vi "Serial Send Characters To Arduino.vi"() -> ()   [LabVIEW 2014]
uses:
  <vilib>/Instr/_visa.llb/VISA Configure Serial Port (Instr).vi
panel:
  in  "stop":bool
  out "error out":errorcluster
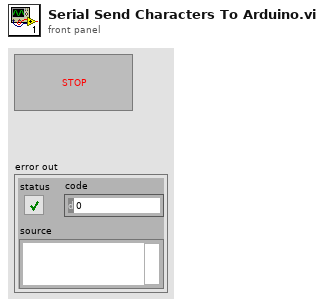
[diagram p1: front panel]
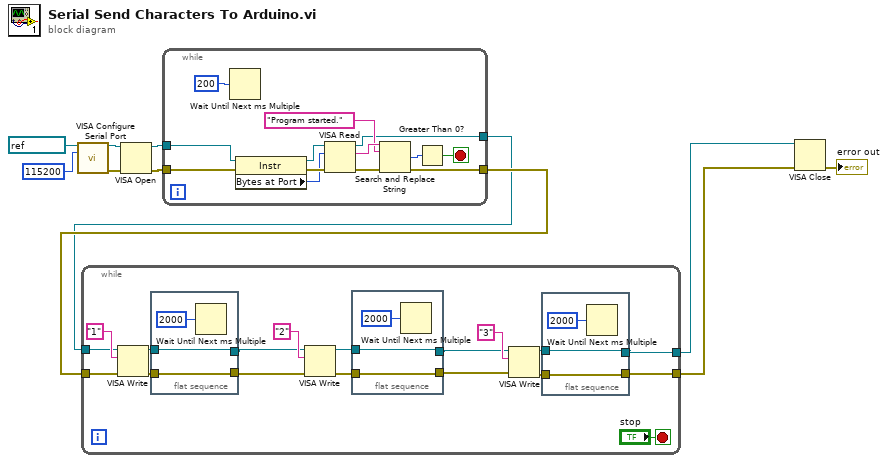
[diagram p0: block diagram]
diagram:
  n1 = call-poly "VISA Configure Serial Port"("VISA resource name"=refnum<visa-resource-name> "COM5", "baud rate (9600)"=u32 115200) -> ("VISA resource name out"=w7:refnum<visa-resource-name>, "error out"=w8:errorcluster)  [unwired: 12 in]
  n2 = VISA Open(error in (no error)=w8, VISA resource name=w7) -> (VISA resource name=w6:refnum<visa-resource-name>, error out=w5:errorcluster)  [unwired: 3 in]
  n3 = while {
    tunnel: w6 -> [w24]
    tunnel: w5 -> [w23]
    tunnel: [w14] -> w4
    tunnel: [w13] -> w3
    stop <- w22 stop-if-true
    n4 = Wait Until Next ms Multiple(millisecond multiple=u32 200) -> ()  [unwired: 1 out]
    n5 = property class="Instr"(reference=w24, error in=w23) -> (reference out=w19:refnum<visa-resource-name>, error out=w20:errorcluster, "Bytes at Port"=w12:u32)
    n6 = VISA Read(VISA resource name=w19, byte count=w12, error in (no error)=w20) -> (VISA resource name out=w13:refnum<visa-resource-name>, read buffer=w18:string, error out=w15:errorcluster)  [unwired: 1 out]
    n7 = Search and Replace String(input string=w18, search string="Program started." ("x"), error in=w15) -> (number of replacements=w16:i32, error out=w14:errorcluster)  [unwired: 5 in, 2 out]
    n8 = Greater Than 0?(x=w16) -> (x > 0?=w22:bool)
  }
  n9 = while {
    tunnel: w4 -> [w41]
    tunnel: w3 -> [w40]
    tunnel: [w26] -> w2
    tunnel: [w25] -> w1
    stop <- "stop" stop-if-true
    n10 = VISA Write(VISA resource name=w40, write buffer="1", error in (no error)=w41) -> (VISA resource name out=w39:refnum<visa-resource-name>, error out=w38:errorcluster)  [unwired: 1 out]
    n11 = flat-sequence {
      tunnel: [w50] -> w28
      tunnel: w39 -> [w50]
      tunnel: [w49] -> w29
      tunnel: w38 -> [w49]
      frame #0 {
        n12 = Wait Until Next ms Multiple(millisecond multiple=u32 2000) -> ()  [unwired: 1 out]
      }
    }
    n13 = VISA Write(VISA resource name=w28, write buffer="2", error in (no error)=w29) -> (VISA resource name out=w36:refnum<visa-resource-name>, error out=w37:errorcluster)  [unwired: 1 out]
    n14 = flat-sequence {
      tunnel: [w47] -> w31
      tunnel: w36 -> [w47]
      tunnel: [w46] -> w30
      tunnel: w37 -> [w46]
      frame #0 {
        n15 = Wait Until Next ms Multiple(millisecond multiple=u32 2000) -> ()  [unwired: 1 out]
      }
    }
    n16 = VISA Write(VISA resource name=w31, write buffer="3", error in (no error)=w30) -> (VISA resource name out=w33:refnum<visa-resource-name>, error out=w32:errorcluster)  [unwired: 1 out]
    n17 = flat-sequence {
      tunnel: [w44] -> w26
      tunnel: w33 -> [w44]
      tunnel: [w43] -> w25
      tunnel: w32 -> [w43]
      frame #0 {
        n18 = Wait Until Next ms Multiple(millisecond multiple=u32 2000) -> ()  [unwired: 1 out]
      }
    }
  }
  n19 = VISA Close(VISA resource name=w2, error in (no error)=w1) -> (error out=→"error out":errorcluster)
